vi "Remember_Results_Files.vi"(1 "Filename to Remember":path) -> (0 "List of Filenames":path[](array[path]))   [LabVIEW 2010]
uses:
  Globals/Meas_global.vi
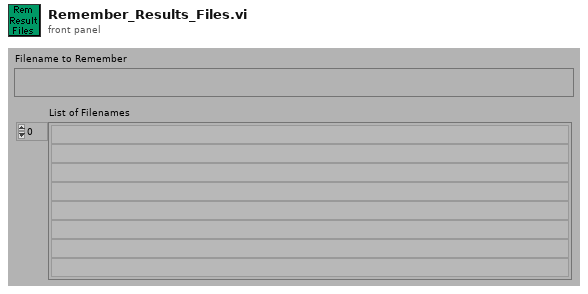
[diagram p1: front panel]
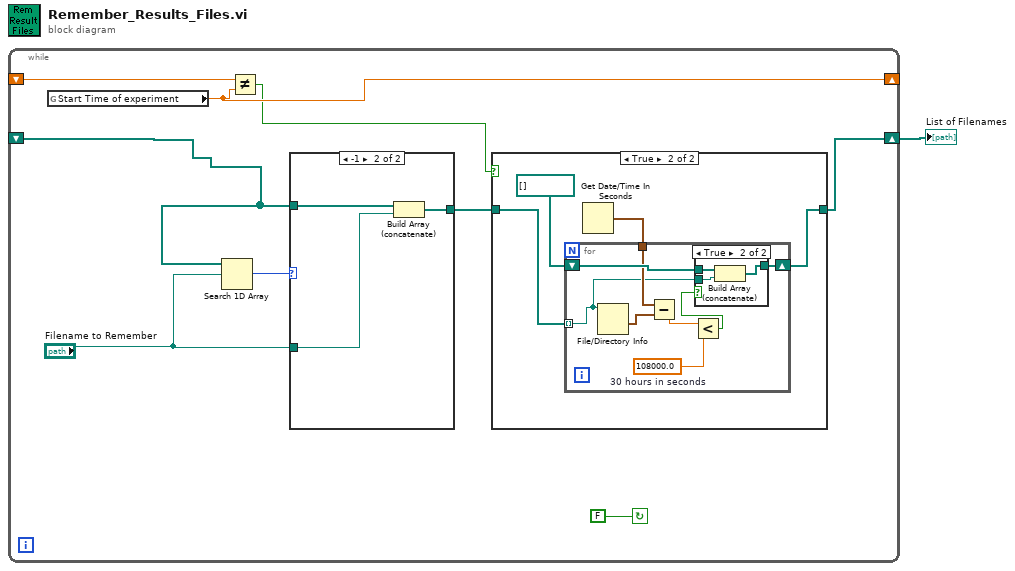
[diagram p0: block diagram]
diagram:
  n1 = while {
    shift-left: _ -> [w7]
    shift-right: [w2] -> w1
    shift-right: [w5] -> _
    shift-left: _ -> [w6]
    stop <- FALSE continue-if-true
    n2 = global read "Meas_global.vi" "Start Time of experiment"() -> (w5:dbl)
    n3 = Search 1D Array(1D array=w7, element="Filename to Remember") -> (index of element=w9:i32)  [unwired: 1 out]
    n4 = Not Equal?(x=w6, y=w5) -> (x != y?=w3:bool)
    n5 = case shown="-1" w9 {
      tunnel: w7 -> [w28 w31]
      tunnel: "Filename to Remember" -> [_ w30]
      tunnel: [w28 w29] -> w4
      frame 0, Default {
      }
      frame -1 {
        n6 = Build Array (concatenate)(w31, w30) -> (w29:path[])
      }
    }
    n7 = case shown="True" w3 {
      tunnel: [w11 w13] -> w2
      tunnel: w4 -> [w11 w15]
      frame False {
      }
      frame True {
        n8 = Get Date/Time In Seconds() -> (seconds since 1Jan1904=w12:timestamp)
        n9 = for {
          tunnel: w15 -> [w17] mode=indexing
          shift-right: [w16] -> w13
          shift-left: path[] [] -> [w23]
          tunnel: w12 -> [w21]
          w19 = 108000.0  # 30 hours in seconds
          n10 = File/Directory Info(path=w17) -> (last mod=w22:timestamp)  [unwired: 1 in, 6 out]
          n11 = Subtract(x=w21, y=w22) -> (x-y=w20:dbl)
          n12 = Less?(x=w20, y=w19) -> (x < y?=w18:bool)
          n13 = case shown="True" w18 {
            tunnel: w23 -> [w24 w27]
            tunnel: w17 -> [_ w26]
            tunnel: [w24 w25] -> w16
            frame False {
            }
            frame True {
              n14 = Build Array (concatenate)(w27, w26) -> (w25:path[])
            }
          }
        }
      }
    }
  }
  "List of Filenames" <- w1
